vi "Read Value (private).vi"(8 "error in (no error)":errorcluster, 9 "timeout in ms (-1)":i32=-1, 11 "Future in":refnum<class "Future.lvclass">) -> (0 "error out":errorcluster, 1 "timed out?":bool, 2 "Value":variant, 3 "Future out":refnum<class "Future.lvclass">)   [LabVIEW 2017, in "Promise Future.lvlib" / "Future.lvclass"]
uses:
  Future.lvclass
  Future.lvclass/Future.ctl
  State/State.lvclass
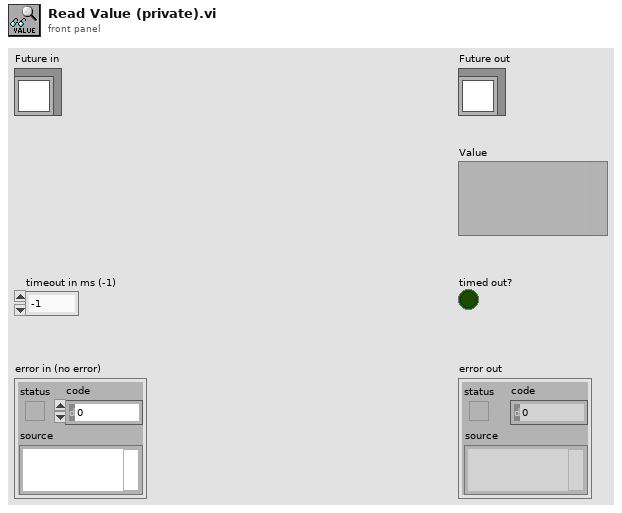
[diagram p1: front panel]
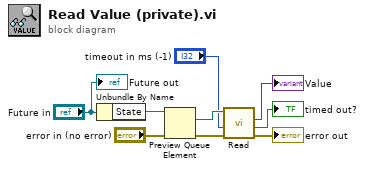
[diagram p0: block diagram]
diagram:
  n1 = Unbundle By Name("Future in") -> ("State"=w8:refnum<queue>)
  n2 = Preview Queue Element(queue=w8, error in (no error)="error in (no error)") -> (element=w6:refnum<class "State.lvclass">, error out=w5:errorcluster)  [unwired: 1 in, 2 out]
  n3 = call "Read.vi"("error in (no error)"=w5, "timeout in ms (-1)"="timeout in ms (-1)", "State in"=w6) -> ("error out"=→"error out":errorcluster, "timed out?"=→"timed out?":bool, "Value"=→"Value":variant)  [unwired: 6 in]
  "Future out" <- "Future in"
